vi "Load Control Values into VI.vi"(8 "error in":errorcluster, 10 "Control Values":T1[](array[typedef]), 11 "VI in":refnum<vi>) -> (0 "error out":errorcluster)   [LabVIEW 2020]
uses:
  <vilib>/addons/analyzer/_analyzerctrls.llb/VIAnCtl Config Control Value.ctl
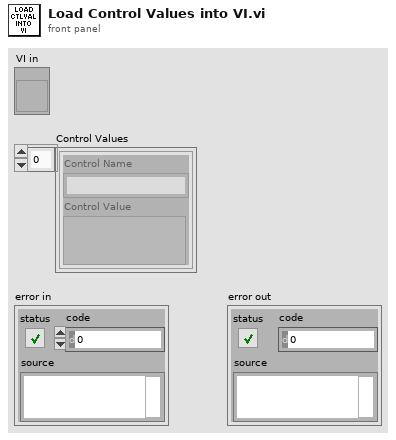
[diagram p1: front panel]
types:
  T1 = typedef "VIAnCtl Config Control Value.ctl" = cluster{"Control Name":string, "Control Value":variant}
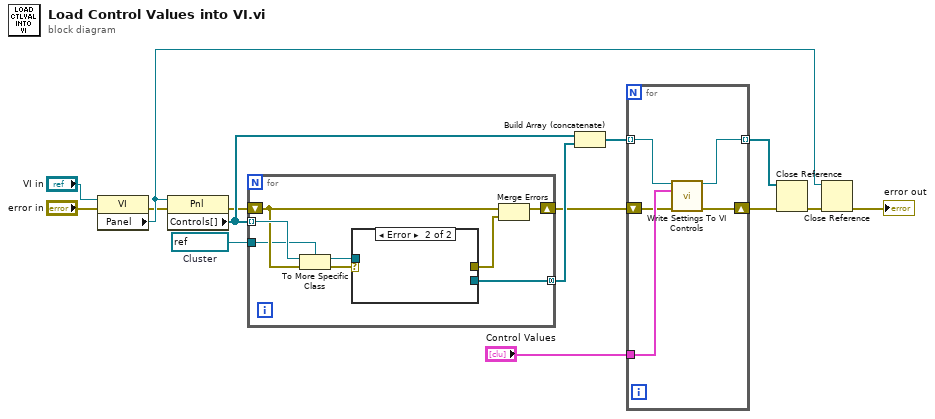
[diagram p0: block diagram]
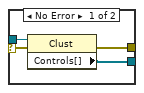
[diagram p2: hidden frame]
diagram:
  w9 = refnum<vi> refnum  # Cluster
  n1 = property class="VI"(reference="VI in", error in="error in") -> (error out=w2:errorcluster, "Panel"=w7:refnum<vi>)  [unwired: 1 out]
  n2 = property class="Pnl"(reference=w7, error in=w2) -> (error out=w3:errorcluster, "Controls[]"=w12:refnum<vi>[])  [unwired: 1 out]
  n3 = for {
    tunnel: w12 -> [w23] mode=indexing
    tunnel: [w20] -> w11 mode=concatenating
    shift-right: [w18] -> w4
    shift-left: w3 -> [w19]
    tunnel: w9 -> [w16]
    n4 = To More Specific Class(target class=w16, reference=w23, error in=w19) -> (specific class reference=w21:refnum<vi>, error out=w22:errorcluster)
    n5 = case shown="Error" w22 {
      selector: w22 -> [w26 _]
      tunnel: w21 -> [w27 _]
      tunnel: [w25 _] -> w20
      tunnel: [w24 _] -> w17
      frame No Error {
        n6 = property class="Clust"(reference=w27, error in=w26) -> (error out=w24:errorcluster, "Controls[]"=w25:refnum<vi>[])  [unwired: 1 out]
      }
      frame Error {
      }
    }
    n7 = Merge Errors(w19, w17) -> (w18:errorcluster)
  }
  n8 = Build Array (concatenate)(w12, w11) -> (w13:refnum<vi>[])
  n9 = for {
    shift-right: [w32] -> w5
    shift-left: w4 -> [w30]
    tunnel: "Control Values" -> [w31]
    tunnel: w13 -> [w29] mode=indexing
    tunnel: [w28] -> w14 mode=indexing
    n10 = call <vilib>:"Write Settings To VI Controls.vi"("Control In"=w29, "Control Values"=w31, "error in"=w30) -> ("Control Out"=w28:refnum<vi>, "error out"=w32:errorcluster)  [unwired: 11 in]
  }
  n11 = Close Reference(reference=w14, error in (no error)=w5) -> (error out=w6:errorcluster)
  n12 = Close Reference(reference=w7, error in (no error)=w6) -> (error out=→"error out":errorcluster)
